vi "ReversedEngineering_GetDiagramComments.vi"(0 "Diagram":refnum<vi>, 2 "CommentsSerachActions":T1, 5 "error in":errorcluster) -> (15 "Comments":string[](array[string]), 19 "error out":errorcluster)   [LabVIEW 2016]
uses:
  <resource>/Framework/Providers/Open_GDS/UML/ReversedEngineering/private/ReversedEngineering StateDiagramCommentSearchType.ctl
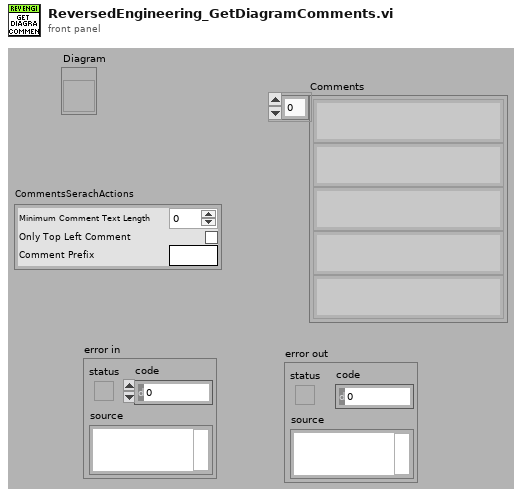
[diagram p1: front panel]
types:
  T1 = typedef "ReversedEngineering StateDiagramCommentSearchType.ctl" = cluster{"MinimumTextLength":i32, "OnlyTopLeftComment":bool, "CommentPrefix":string}
  T2 = typedef "LVPositionTypeDef.ctl" = cluster{"Left":i32, "Top":i32}
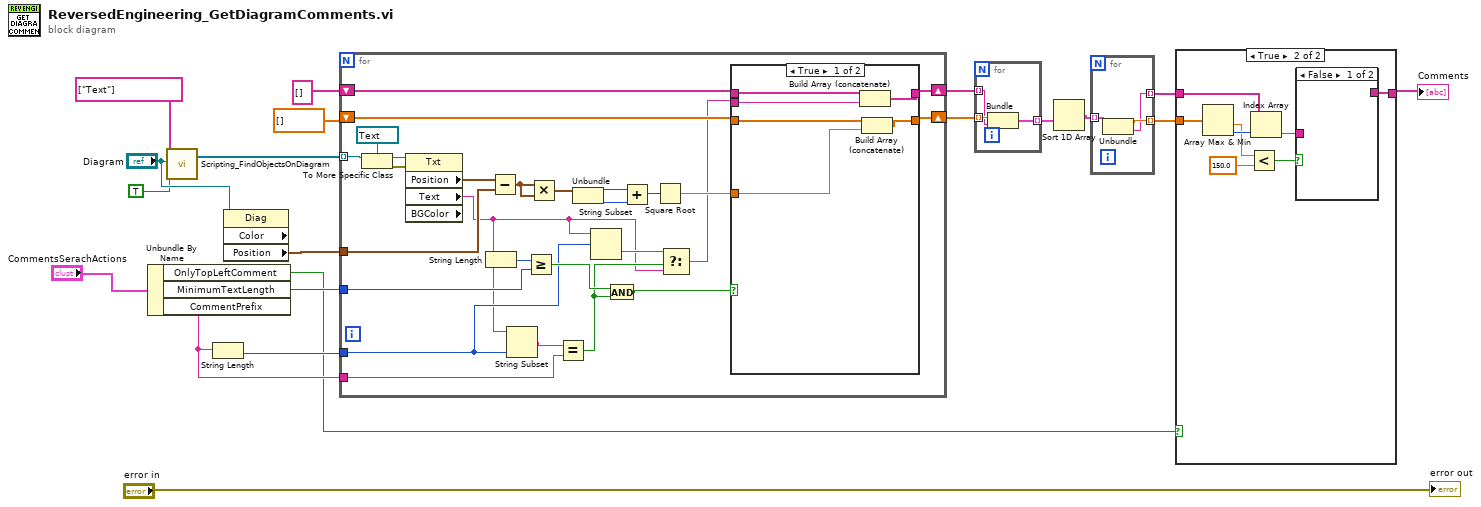
[diagram p0: block diagram]
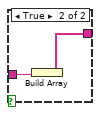
[diagram p3: hidden frame]
diagram:
  n1 = Unbundle By Name("CommentsSerachActions") -> ("OnlyTopLeftComment"=w9:bool, "MinimumTextLength"=w17:i32, "CommentPrefix"=w11:string)
  n2 = call <resource>:"Scripting_FindObjectsOnDiagram.vi"("NodeTypesToSearchFor"=string[] ["Text"], "Diagram(Ignored If Not Wired)"="Diagram", "Don'tSearchSubStructures(False)"=TRUE) -> ("Nodes"=w15:refnum<vi>[])  [unwired: 15 in, 1 out]
  n3 = String Length(string=w11) -> (length=w12:i32)
  n4 = property class="Diag" props=["Color", "Position"](reference="Diagram") -> ("Position"=w13:T2)  [unwired: 1 in, 3 out]
  n5 = for {
    shift-right: [w47] -> w5
    shift-left: string[] [] ("StateActions") -> [w46]
    tunnel: w17 -> [w40]
    tunnel: w15 -> [w33] mode=indexing
    shift-right: [w35] -> w6
    shift-left: dbl[] [] -> [w36]
    tunnel: w13 -> [w31]
    tunnel: w12 -> [w24]
    tunnel: w11 -> [w38]
    n6 = To More Specific Class(target class=refnum<vi> refnum ("Diagram(Ignored If Not Wired)"), reference=w33) -> (specific class reference=w43:refnum<vi>, error out=w44:errorcluster)  [unwired: 1 in]
    n7 = property class="Txt" props=["Position", "Text", "BGColor"](reference=w43, error in=w44) -> ("Position"=w32:T2, "Text"=w22:string)  [unwired: 3 out]
    n8 = String Length(string=w22) -> (length=w41:i32)
    n9 = Subtract(x=w32, y=w31) -> (x-y=w30:T2)
    n10 = String Subset(string=w22, length (rest)=w24) -> (substring=w39:string)  [unwired: 1 in]
    n11 = Greater Or Equal?(x=w41, y=w40) -> (x >= y?=w37:bool)
    n12 = Multiply(x=w30, y=w30) -> (x*y=w29:T2)
    n13 = Equal?(x=w39, y=w38) -> (x = y?=w25:bool)
    n14 = Unbundle(w29) -> ("Left"=w28:i32, "Top"=w27:i32)
    n15 = String Subset(string=w22, offset (0)=w24) -> (substring=w23:string)  [unwired: 1 in]
    n16 = And(x=w37, y=w25) -> (x .and. y?=w26:bool)
    n17 = Add(x=w28, y=w27) -> (x+y=w45:i32)
    n18 = Square Root(x=w45) -> (sqrt(x)=w34:dbl)
    n19 = Select(t=w23, s=w25, f=w22) -> (s? t:f=w21:string)
    n20 = case shown="True" w26 {
      tunnel: w46 -> [w53 w55]
      tunnel: [w52 w55] -> w47
      tunnel: w21 -> [w51 _]
      tunnel: w36 -> [w50 w54]
      tunnel: [w49 w54] -> w35
      tunnel: w34 -> [w48 _]
      frame True {
        n21 = Build Array (concatenate)(w53, w51) -> (w52:string[])
        n22 = Build Array (concatenate)(w50, w48) -> (w49:dbl[])
      }
      frame False {
        # "Ignored"
      }
    }
  }
  n23 = for {
    tunnel: w6 -> [w58] mode=indexing
    tunnel: w5 -> [w57] mode=indexing
    tunnel: [w56] -> w4 mode=indexing
    n24 = Bundle(w58, w57) -> (w56:cluster{dbl, string})  [unwired: 1 in]
  }
  n25 = Sort 1D Array(array=w4) -> (sorted array=w3:cluster{dbl, string}[])
  n26 = for {
    tunnel: w3 -> [w61] mode=indexing
    tunnel: [w60] -> w2 mode=indexing
    tunnel: [w59] -> w1 mode=indexing
    n27 = Unbundle(w61) -> (w60:dbl, w59:string)
  }
  n28 = case shown="True" w9 {
    tunnel: w1 -> [w62 w69]
    tunnel: [w62 w64] -> w8
    tunnel: w2 -> [_ w70]
    frame False {
    }
    frame True {
      n29 = Array Max & Min(array=w70) -> (min value=w67:dbl, min index (indices)=w68:i32)  [unwired: 2 out]
      n30 = Less?(x=w67, y=150.0) -> (x < y?=w65:bool)
      n31 = Index Array(array=w69, index=w68) -> (element=w63:string)
      n32 = case shown="False" w65 {
        tunnel: [_ w71] -> w64
        tunnel: w63 -> [_ w72]
        frame False {
        }
        frame True {
          n33 = Build Array(w72) -> (w71:string[])
        }
      }
    }
  }
  "Comments" <- w8
  "error out" <- "error in"
